vi "DER SetpointP.vi"(8 "error in":errorcluster, 10 "DER_SetPointP":T1, 11 "SCADA in":refnum<class "EMS.lvclass">) -> (0 "error out":errorcluster, 3 "SCADA out":refnum<class "EMS.lvclass">)   [LabVIEW 2018, in "EMS Core.lvlib" / "EMS.lvclass"]
uses:
  EMS.lvclass
  C:/Users/Administrator/Desktop/LabVIEW EMS/EMS Generic Actor/EMS Generic/EMS Generic.lvclass
  <vilib>/ORNL/CSEISMIC DDS/CSEISMIC DDS Base/Data Types/DER_SetPointP.ctl
  <vilib>/ORNL/CSEISMIC DDS/CSEISMIC DDS Base/Data Types/Controls/DeviceID.ctl
  EMS.lvclass/EMS.ctl
  IED Actors/DER Actor/DER Messages/Write DER SetpointP Msg/Write DER SetpointP Msg.lvclass/Write DER SetpointP Msg.ctl
  <vilib>/ActorFramework/Message Enqueuer/Message Enqueuer.lvclass/Message Enqueuer.ctl
  <vilib>/ActorFramework/Message Enqueuer/Enqueue.vi
  IED Actors/DER Actor/DER Messages/Write DER SetpointP Msg/Write DER SetpointP Msg.lvclass
  C:/Program Files (x86)/National Instruments/LabVIEW 2018/vi.lib/ActorFramework/Message/Message.lvclass
  <vilib>/ActorFramework/Message Priority Queue/Priority Enqueue.vi
  EMS Generic Actor/EMS Generic/EMS Generic.lvclass
  <vilib>/ORNL/CSEISMIC DDS/CSEISMIC DDS Base/CSEISMIC DDS.lvclass
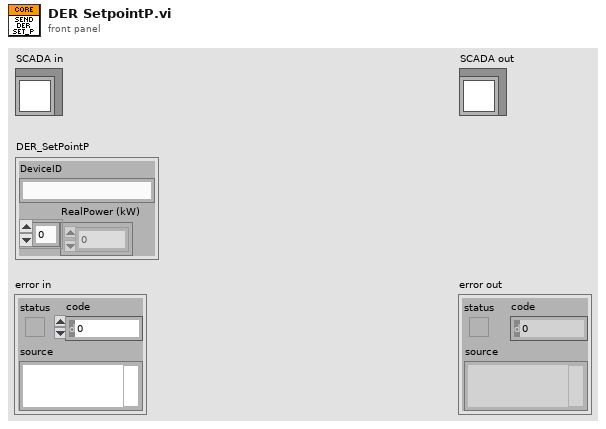
[diagram p1: front panel]
types:
  T1 = typedef "CSEISMIC DDS.lvlib/CSEISMIC DDS.lvclass/DER_SetPointP.ctl" = cluster{"DeviceID":T2, "RealPower (kW)":dbl[]}
  T2 = typedef "CSEISMIC DDS.lvlib/CSEISMIC DDS.lvclass/DeviceID.ctl" = string
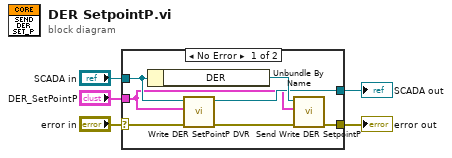
[diagram p0: block diagram]
diagram:
  n1 = case shown="No Error" "error in" {
    selector: "error in" -> [w7 w14]
    tunnel: [w11 w14] -> w4
    tunnel: [w9 w13] -> w2
    tunnel: "SCADA in" -> [w10 w13]
    tunnel: "DER_SetPointP" -> [w8 _]
    frame No Error {
      n2 = Unbundle By Name(w10) -> ("DER"=w12:refnum<class "Message Enqueuer.lvclass">)
      n3 = call "Write DER SetPointP DVR.vi"("error in"=w7, "DER_SetPointP"=w8, "EMS Generic in"=w10) -> ("error out"=w6:errorcluster, "EMS Generic out"=w9:refnum<class "EMS.lvclass">)  [unwired: 7 in]
      n4 = call "Send Write DER SetpointP.vi"("error in (no error)"=w6, "DER_SetPointP"=w8, "Message Enqueuer"=w12) -> ("error out"=w11:errorcluster)  [unwired: 7 in, 1 out]
    }
    frame Error {
    }
  }
  "error out" <- w4
  "SCADA out" <- w2
